vi "Global_MessageBits.vi"() -> ()   [LabVIEW 2013]
panel:
  out "M_Bits":i8[](array[numeric])
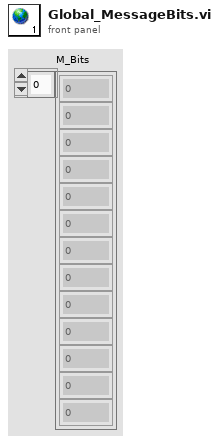
[diagram p1: front panel]
diagram:
